vi "Write Single Coil Request.vi"(8 "error in (no error)":errorcluster, 9 "coil value":bool, 10 "starting address":u16) -> (0 "error out":errorcluster, 2 "Modbus data unit out":refnum<class "Modbus Data Unit (PDU).lvclass">)   [LabVIEW 2020, in "SubVIs.lvlib" / "Master Function Definition.lvlib"]
doc: "This VI forms a modbus data unit for writing a single coil."
uses:
  <vilib>/Modbus/subvis/Data and Functions/Master Function Definition/Master Function Definition.lvlib
  <vilib>/Modbus/subvis/Modbus Data Unit (PDU)/Modbus Data Unit (PDU).lvclass
  <vilib>/Modbus/subvis/Modbus Data Unit (PDU)/Modbus Data Unit (PDU).lvclass/Modbus Data Unit (PDU).ctl
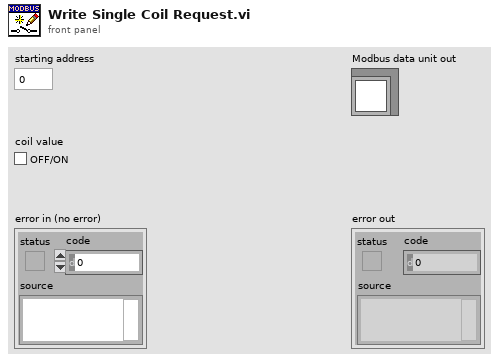
[diagram p1: front panel]
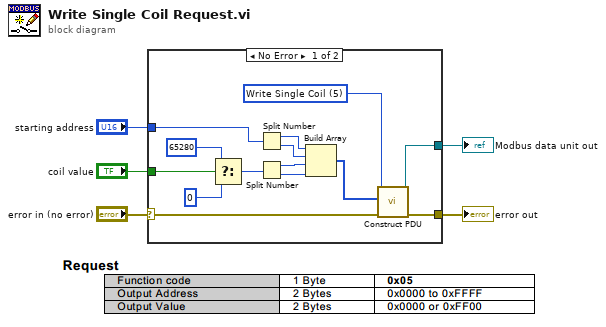
[diagram p0: block diagram]
diagram:
  n1 = case shown="No Error" "error in (no error)" {
    selector: "error in (no error)" -> [w6 w20]
    tunnel: [w19 w20] -> w5
    tunnel: "starting address" -> [w18 _]
    tunnel: [w17 _] -> w3
    tunnel: "coil value" -> [w10 _]
    frame No Error {
      w11 = u8 5 items=["Read Discrete Inputs"=2, "Read Coils"=1, "Write Single Coil"=5, "Write Multiple Coils"=15, "Read Input Register"=4, "Read Holding Registers"=3, "Write Single Register"=6, "Write Multiple Registers"=16, "Read/Write Multiple Registers"=23, "Mask Write Register"=22, "Read FIFO Queue"=24, "Read File Record"=20, "Write File Record"=21, "Read Exception Status"=7, "Diagnostic"=8, "Get Com Event Counter"=11, "Get Com Event Log"=12, "Report Slave ID"=17, "Read Device Identification"=43] ("Function")
      n2 = Select(t=u16 65280 ("y"), s=w10, f=u16 0 ("y")) -> (s? t:f=w7:u16)
      n3 = Split Number(x=w18) -> (hi(x)=w13:u8, lo(x)=w14:u8)
      n4 = Split Number(x=w7) -> (hi(x)=w15:u8, lo(x)=w16:u8)
      n5 = Build Array(w13, w14, w15, w16) -> (w12:u8[])
      n6 = call <vilib>:"Construct PDU.vi"("error in (no error)"=w6, "data"=w12, "function"=w11) -> ("error out"=w19:errorcluster, "Modbus data unit out"=w17:refnum<class "Modbus Data Unit (PDU).lvclass">)  [unwired: 7 in]
    }
    frame Error {
    }
  }
  "error out" <- w5
  "Modbus data unit out" <- w3
